vi "test_read-nmea-data2.vi"() -> ()   [LabVIEW 2019] (continued)
308,,2*7E\n\t\n15:10:22.66\tF9P\t$GBGSV,1,1,03,11,50,131,19,14,87,138,20,33,60,219,20,1*47\n\t\n15:10:22.68\tF9P\t$GBGSV,1,1,03,11,50,131,,14,87,138,22,33,60,219,,3*4D\n\t\n15:10:22.70\tF9P\t$GNGLL,3723.57293,N,12656.88370,E,061024.00,A,A*7B\n\t\n15:10:22.72\tF9P\t\t\n15:10:22.74\tF9P\t\t\n15:10:22.76\tF9P\t\t\n15:10:22.78\tF9P\t\t\n15:10:22.80\tF9P\t\t\n15:10:22.82\tF9P\t\t\n15:10:22.84\tF9P\t\t\n15:10:22.86\tF9P\t\t\n15:10:22.88\tF9P\t\t\n15:10:22.90\tF9P\t\t\n15:10:22.92\tF9P\t\t\n15:10:22.94\tF9P\t\t\n15:10:22.96\tF9P\t\t\n15:10:22.98\tF9P\t\t\n15:10:23.00\tF9P\t\t\n15:10:23.02\tF9P\t\t\n15:10:23.04\tF9P\t\t\n15:10:23.06\tF9P\t\t\n15:10:23.08\tF9P\t\t\n15:10:23.10\tF9P\t\t\n15:10:23.12\tF9P\t\t\n15:10:23.14\tF9P\t\t\n15:10:23.16\tF9P\t\t\n15:10:23.18\tF9P\t\t\n15:10:23.20\tF9P\t\t\n15:10:23.22\tF9P\t\t\n15:10:23.24\tF9P\t$GNRMC,061025.00,A,3723.57257,N,12656.88383,E,0.634,,250720,,,A,V*1E\n\t\n15:10:23.26\tF9P\t$GNVTG,,T,,M,0.634,N,1.174,K,A*3F\n\t\n15:10:23.28\tF9P\t$GNGGA,061025.00,3723.57257,N,12656.88383,E,1,12,0.64,59.6,M,18.5,M,,*7C\n\t\n15:10:23.30\tF9P\t$GNGSA,A,3,12,06,19,05,17,09,04,02,,,,,1.19,0.64,1.00,1*0A\n\t\n15:10:23.32\tF9P\t$GNGSA,A,3,85,71,84,,,,,,,,,,1.19,0.64,1.00,2*0F\n\t\n15:10:23.34\tF9P\t$GNGSA,A,3,36,19,11,04,09,12,,,,,,,1.19,0.64,1.00,3*0A\n\t\n15:10:23.36\tF9P\t$GNGSA,A,3,14,11,33,,,,,,,,,,1.19,0.64,1.00,4*0B\n\t\n15:10:23.38\tF9P\t$GPGSV,3,1,09,02,54,318,21,04,19,044,12,05,36,246,24,06,65,046,25,1*6C\n\t\n15:10:23.40\tF9P\t$GPGSV,3,2,09,09,45,075,26,12,24,278,19,17,34,153,21,19,53,156,23,1*6A\n\t\n15:10:23.42\tF9P\t$GPGSV,3,3,09,25,12,307,12,1*5E\n\t\n15:10:23.44\tF9P\t$GPGSV,3,1,09,02,54,318,,04,19,044,,05,36,246,18,06,65,046,15,6*67\n\t\n15:10:23.46\tF9P\t$GPGSV,3,2,09,09,45,075,,12,24,278,,17,34,153,,19,53,156,,6*63\n\t\n15:10:23.48\tF9P\t$GPGSV,3,3,09,25,12,307,,6*5A\n\t\n15:10:23.50\tF9P\t$GLGSV,2,1,08,69,12,031,,70,72,041,,71,51,205,17,72,03,209,,1*74\n\t\n15:10:23.52\tF9P\t$GLGSV,2,2,08,77,01,326,,84,20,122,09,85,70,065,19,86,36,330,,1*7A\n\t\n15:10:23.54\tF9P\t$GLGSV,2,1,08,69,12,031,,70,72,041,,71,51,205,18,72,03,209,,3*79\n\t\n15:10:23.56\tF9P\t$GLGSV,2,2,08,77,01,326,,84,20,122,09,85,70,065,19,86,36,330,,3*78\n\t\n15:10:23.58\tF9P\t$GAGSV,2,1,08,02,09,298,09,04,66,119,25,09,31,193,17,11,71,357,25,7*75\n\t\n15:10:23.60\tF9P\t$GAGSV,2,2,08,12,40,102,09,19,27,045,21,25,09,249,,36,25,308,13,7*73\n\t\n15:10:23.62\tF9P\t$GAGSV,2,1,08,02,09,298,,04,66,119,,09,31,193,19,11,71,357,11,2*77\n\t\n15:10:23.64\tF9P\t$GAGSV,2,2,08,12,40,102,,19,27,045,,25,09,249,,36,25,308,,2*7E\n\t\n15:10:23.66\tF9P\t$GBGSV,1,1,03,11,50,131,19,14,87,138,21,33,60,219,21,1*47\n\t\n15:10:23.68\tF9P\t$GBGSV,1,1,03,11,50,131,,14,87,138,23,33,60,219,,3*4C\n\t\n15:10:23.70\tF9P\t$GNGLL,3723.57257,N,12656.88383,E,061025.00,A,A*7E\n\t\n15:10:23.72\tF9P\t\t\n15:10:23.74\tF9P\t\t\n15:10:23.76\tF9P\t\t\n15:10:23.78\tF9P\t\t\n15:10:23.80\tF9P\t\t\n15:10:23.82\tF9P\t\t\n15:10:23.84\tF9P\t\t\n15:10:23.86\tF9P\t\t\n15:10:23.88\tF9P\t\t\n15:10:23.90\tF9P\t\t\n15:10:23.92\tF9P\t\t\n15:10:23.95\tF9P\t\t\n15:10:23.97\tF9P\t\t\n15:10:23.99\tF9P\t\t\n15:10:24.01\tF9P\t\t\n15:10:24.03\tF9P\t\t\n15:10:24.05\tF9P\t\t\n15:10:24.07\tF9P\t\t\n15:10:24.09\tF9P\t\t\n15:10:24.11\tF9P\t\t\n15:10:24.13\tF9P\t\t\n15:10:24.15\tF9P\t\t\n15:10:24.17\tF9P\t\t\n15:10:24.19\tF9P\t\t\n15:10:24.21\tF9P\t\t\n15:10:24.23\tF9P\t\t\n15:10:24.25\tF9P\t$GNRMC,061026.00,A,3723.57217,N,12656.88385,E,0.897,,250720,,,A,V*18\n\t\n15:10:24.27\tF9P\t$GNVTG,,T,,M,0.897,N,1.661,K,A*3B\n\t\n15:10:24.29\tF9P\t$GNGGA,061026.00,3723.57217,N,12656.88385,E,1,12,0.64,59.8,M,18.5,M,,*73\n\t\n15:10:24.31\tF9P\t$GNGSA,A,3,12,06,19,05,17,09,04,02,,,,,1.19,0.64,1.00,1*0A\n\t\n15:10:24.33\tF9P\t$GNGSA,A,3,85,71,84,,,,,,,,,,1.19,0.64,1.00,2*0F\n\t\n15:10:24.35\tF9P\t$GNGSA,A,3,36,19,11,04,09,12,,,,,,,1.19,0.64,1.00,3*0A\n\t\n15:10:24.37\tF9P\t$GNGSA,A,3,14,11,33,,,,,,,,,,1.19,0.64,1.00,4*0B\n\t\n15:10:24.39\tF9P\t$GPGSV,3,1,09,02,54,318,23,04,19,044,11,05,36,246,25,06,65,046,30,1*68\n\t\n15:10:24.41\tF9P\t$GPGSV,3,2,09,09,45,075,27,12,24,278,20,17,34,153,24,19,53,156,21,1*66\n\t\n15:10:24.43\tF9P\t$GPGSV,3,3,09,25,12,307,13,1*5F\n\t\n15:10:24.45\tF9P\t$GPGSV,3,1,09,02,54,318,,04,19,044,,05,36,246,17,06,65,046,16,6*6B\n\t\n15:10:24.47\tF9P\t$GPGSV,3,2,09,09,45,075,19,12,24,278,,17,34,153,,19,53,156,,6*6B\n\t\n15:10:24.49\tF9P\t$GPGSV,3,3,09,25,12,307,,6*5A\n\t\n15:10:24.51\tF9P\t$GLGSV,2,1,08,69,12,031,,70,72,041,,71,51,205,16,72,03,209,,1*75\n\t\n15:10:24.53\tF9P\t$GLGSV,2,2,08,77,01,326,,84,20,122,09,85,70,065,19,86,36,330,,1*7A\n\t\n15:10:24.55\tF9P\t$GLGSV,2,1,08,69,12,031,,70,72,041,,71,51,205,18,72,03,209,,3*79\n\t\n15:10:24.57\tF9P\t$GLGSV,2,2,08,77,01,326,,84,20,122,10,85,70,065,19,86,36,330,,3*70\n\t\n15:10:24.59\tF9P\t$GAGSV,2,1,08,02,09,298,09,04,66,119,25,09,31,193,18,11,71,357,25,7*7A\n\t\n15:10:24.61\tF9P\t$GAGSV,2,2,08,12,40,102,10,19,27,045,20,25,09,249,,36,25,308,13,7*7A\n\t\n15:10:24.63\tF9P\t$GAGSV,2,1,08,02,09,298,,04,66,119,,09,31,193,20,11,71,357,09,2*74\n\t\n15:10:24.65\tF9P\t$GAGSV,2,2,08,12,40,102,,19,27,045,,25,09,249,,36,25,308,,2*7E\n\t\n15:10:24.67\tF9P\t$GBGSV,1,1,03,11,50,131,21,14,87,138,20,33,60,219,20,1*4C\n\t\n15:10:24.69\tF9P\t$GBGSV,1,1,03,11,50,131,,14,87,138,23,33,60,219,,3*4C\n\t\n15:10:24.71\tF9P\t$GNGLL,3723.57217,N,12656.88385,E,061026.00,A,A*7F\n\t\n15:10:24.73\tF9P\t\t\n15:10:24.75\tF9P\t\t\n15:10:24.77\tF9P\t\t\n15:10:24.79\tF9P\t\t\n15:10:24.81\tF9P\t\t\n15:10:24.83\tF9P\t\t\n15:10:24.85\tF9P\t\t\n15:10:24.87\tF9P\t\t\n15:10:24.89\tF9P\t\t\n15:10:24.91\tF9P\t\t\n15:10:24.93\tF9P\t\t\n15:10:24.95\tF9P\t\t\n15:10:24.97\tF9P\t\t\n15:10:24.99\tF9P\t\t\n15:10:25.01\tF9P\t\t\n15:10:25.03\tF9P\t\t\n15:10:25.05\tF9P\t\t\n15:10:25.07\tF9P\t\t\n15:10:25.09\tF9P\t\t\n15:10:25.11\tF9P\t\t\n15:10:25.13\tF9P\t\t\n15:10:25.15\tF9P\t\t\n15:10:25.17\tF9P\t\t\n15:10:25.19\tF9P\t\t\n15:10:25.21\tF9P\t\t\n15:10:25.23\tF9P\t\t\n15:10:25.25\tF9P\t$GNRMC,061027.00,A,3723.57149,N,12656.88411,E,2.245,169.19,250720,,,A,V*04\n\t\n15:10:25.27\tF9P\t$GNVTG,169.19,T,,M,2.245,N,4.158,K,A*2C\n\t\n15:10:25.29\tF9P\t$GNGGA,061027.00,3723.57149,N,12656.88411,E,1,12,0.64,59.6,M,18.5,M,,*7E\n\t\n15:10:25.31\tF9P\t$GNGSA,A,3,12,06,19,05,17,09,04,02,,,,,1.19,0.64,1.00,1*0A\n\t\n15:10:25.33\tF9P\t$GNGSA,A,3,85,71,84,,,,,,,,,,1.19,0.64,1.00,2*0F\n\t\n15:10:25.35\tF9P\t$GNGSA,A,3,36,19,11,04,09,12,,,,,,,1.19,0.64,1.00,3*0A\n\t\n15:10:25.37\tF9P\t$GNGSA,A,3,14,11,33,,,,,,,,,,1.19,0.64,1.00,4*0B\n\t\n15:10:25.39\tF9P\t$GPGSV,3,1,09,02,54,318,23,04,19,044,08,05,36,246,26,06,65,046,22,1*60\n\t\n15:10:25.41\tF9P\t$GPGSV,3,2,09,09,45,075,26,12,24,278,23,17,34,153,23,19,53,156,22,1*60\n\t\n15:10:25.43\tF9P\t$GPGSV,3,3,09,25,12,307,14,1*58\n\t\n15:10:25.45\tF9P\t$GPGSV,3,1,09,02,54,318,,04,19,044,,05,36,246,19,06,65,046,16,6*65\n\t\n15:10:25.47\tF9P\t$GPGSV,3,2,09,09,45,075,18,12,24,278,,17,34,153,20,19,53,156,,6*68\n\t\n15:10:25.49\tF9P\t$GPGSV,3,3,09,25,12,307,,6*5A\n\t\n15:10:25.51\tF9P\t$GLGSV,2,1,08,69,12,031,,70,72,041,,71,51,205,16,72,03,209,,1*75\n\t\n15:10:25.53\tF9P\t$GLGSV,2,2,08,77,01,326,,84,20,122,12,85,70,065,20,86,36,330,,1*7A\n\t\n15:10:25.55\tF9P\t$GLGSV,2,1,08,69,12,031,,70,72,041,,71,51,205,18,72,03,209,,3*79\n\t\n15:10:25.57\tF9P\t$GLGSV,2,2,08,77,01,326,,84,20,122,09,85,70,065,18,86,36,330,,3*79\n\t\n15:10:25.59\tF9P\t$GAGSV,2,1,08,02,09,298,07,04,66,119,26,09,31,193,17,11,71,357,25,7*78\n\t\n15:10:25.61\tF9P\t$GAGSV,2,2,08,12,40,102,12,19,27,045,21,25,09,249,,36,25,308,13,7*79\n\t\n15:10:25.63\tF9P\t$GAGSV,2,1,08,02,09,298,,04,66,119,,09,31,193,19,11,71,357,08,2*7F\n\t\n15:10:25.65\tF9P\t$GAGSV,2,2,08,12,40,102,,19,27,045,,25,09,249,,36,25,308,,2*7E\n\t\n15:10:25.67\tF9P\t$GBGSV,1,1,03,11,50,131,22,14,87,138,22,33,60,219,21,1*4C\n\t\n15:10:25.69\tF9P\t$GBGSV,1,1,03,11,50,131,,14,87,138,22,33,60,219,,3*4D\n\t\n15:10:25.71\tF9P\t$GNGLL,3723.57149,N,12656.88411,E,061027.00,A,A*7C\n\t\n15:10:25.73\tF9P\t\t\n15:10:25.75\tF9P\t\t\n15:10:25.77\tF9P\t\t\n15:10:25.79\tF9P\t\t\n15:10:25.81\tF9P\t\t\n15:10:25.83\tF9P\t\t\n15:10:25.85\tF9P\t\t\n15:10:25.87\tF9P\t\t\n15:10:25.89\tF9P\t\t\n15:10:25.91\tF9P\t\t\n15:10:25.93\tF9P\t\t\n15:10:25.95\tF9P\t\t\n15:10:25.97\tF9P\t\t\n15:10:25.99\tF9P\t\t\n15:10:26.01\tF9P\t\t\n15:10:26.03\tF9P\t\t\n15:10:26.05\tF9P\t\t\n15:10:26.07\tF9P\t\t\n15:10:26.09\tF9P\t\t\n15:10:26.11\tF9P\t\t\n15:10:26.13\tF9P\t\t\n15:10:26.15\tF9P\t\t\n15:10:26.17\tF9P\t\t\n15:10:26.19\tF9P\t\t\n15:10:26.21\tF9P\t\t\n15:10:26.23\tF9P\t\t\n15:10:26.25\tF9P\t$GNRMC,061028.00,A,3723.57082,N,12656.88425,E,1.515,,250720,,,A,V*13\n\t\n15:10:26.27\tF9P\t$GNVTG,,T,,M,1.515,N,2.806,K,A*31\n\t\n15:10:26.29\tF9P\t$GNGGA,061028.00,3723.57082,N,12656.88425,E,1,12,0.64,61.5,M,18.5,M,,*78\n\t\n15:10:26.31\tF9P\t$GNGSA,A,3,12,06,19,05,17,09,04,02,,,,,1.18,0.64,1.00,1*0B\n\t\n15:10:26.33\tF9P\t$GNGSA,A,3,85,71,84,,,,,,,,,,1.18,0.64,1.00,2*0E\n\t\n15:10:26.35\tF9P\t$GNGSA,A,3,36,19,11,04,09,12,,,,,,,1.18,0.64,1.00,3*0B\n\t\n15:10:26.37\tF9P\t$GNGSA,A,3,14,11,33,,,,,,,,,,1.18,0.64,1.00,4*0A\n\t\n15:10:26.39\tF9P\t$GPGSV,3,1,09,02,54,318,22,04,19,044,12,05,36,246,26,06,65,046,23,1*6B\n\t\n15:10:26.41\tF9P\t$GPGSV,3,2,09,09,45,075,25,12,24,278,22,17,34,153,23,19,53,156,23,1*63\n\t\n15:10:26.43\tF9P\t$GPGSV,3,3,09,25,12,307,12,1*5E\n\t\n15:10:26.45\tF9P\t$GPGSV,3,1,09,02,54,318,,04,19,044,,05,36,246,19,06,65,046,15,6*66\n\t\n15:10:26.47\tF9P\t$GPGSV,3,2,09,09,45,075,17,12,24,278,,17,34,153,19,19,53,156,,6*6D\n\t\n15:10:26.49\tF9P\t$GPGSV,3,3,09,25,12,307,,6*5A\n\t\n15:10:26.51\tF9P\t$GLGSV,2,1,08,69,12,031,,70,72,041,,71,51,205,15,72,03,209,,1*76\n\t\n15:10:26.53\tF9P\t$GLGSV,2,2,08,77,01,326,,84,20,122,09,85,70,065,22,86,36,330,,1*72\n\t\n15:10:26.55\tF9P\t$GLGSV,2,1,08,69,12,031,,70,72,041,,71,51,205,17,72,03,209,,3*76\n\t\n15:10:26.57\tF9P\t$GLGSV,2,2,08,77,01,326,,84,20,122,13,85,70,065,18,86,36,330,,3*72\n\t\n15:10:26.59\tF9P\t$GAGSV,2,1,08,02,09,298,10,04,66,119,24,09,31,193,17,11,71,357,25,7*7C\n\t\n15:10:26.61\tF9P\t$GAGSV,2,2,08,12,40,102,13,19,27,045,28,25,09,249,,36,25,308,12,7*70\n\t\n15:10:26.63\tF9P\t$GAGSV,2,1,08,02,09,298,,04,66,119,,09,31,193,19,11,71,357,,2*77\n\t\n15:10:26.65\tF9P\t$GAGSV,2,2,08,12,40,102,,19,27,045,,25,09,249,,36,25,308,,2*7E\n\t\n15:10:26.67\tF9P\t$GBGSV,1,1,03,11,50,131,21,14,87,138,21,33,60,219,21,1*4C\n\t\n15:10:26.69\tF9P\t$GBGSV,1,1,03,11,50,131,,14,87,138,22,33,60,219,,3*4D\n\t\n15:10:26.71\tF9P\t$GNGLL,3723.57082,N,12656.88425,E,061028.00,A,A*72\n\t\n15:10:26.73\tF9P\t\t\n15:10:26.75\tF9P\t\t\n15:10:26.77\tF9P\t\t\n15:10:26.79\tF9P\t\t\n15:10:26.81\tF9P\t\t\n15:10:26.83\tF9P\t\t\n15:10:26.85\tF9P\t\t\n15:10:26.87\tF9P\t\t\n15:10:26.89\tF9P\t\t\n15:10:26.91\tF9P\t\t\n15:10:26.93\tF9P\t\t\n15:10:26.95\tF9P\t\t\n15:10:26.97\tF9P\t\t\n15:10:26.99\tF9P\t\t\n15:10:27.01\tF9P\t\t\n15:10:27.03\tF9P\t\t\n15:10:27.05\tF9P\t\t\n15:10:27.07\tF9P\t\t\n15:10:27.09\tF9P\t\t\n15:10:27.11\tF9P\t\t\n15:10:27.13\tF9P\t\t\n15:10:27.15\tF9P\t\t\n15:10:27.17\tF9P\t\t\n15:10:27.19\tF9P\t\t\n15:10:27.21\tF9P\t\t\n15:10:27.23\tF9P\t\t\n15:10:27.25\tF9P\t$GNRMC,061029.00,A,3723.57008,N,12656.88462,E,2.453,165.29,250720,,,A,V*04\n\t\n15:10:27.27\tF9P\t$GNVTG,165.29,T,,M,2.453,N,4.543,K,A*2C\n\t\n15:10:27.29\tF9P\t$GNGGA,061029.00,3723.57008,N,12656.88462,E,1,12,0.64,62.2,M,18.5,M,,*7C\n\t\n15:10:27.31\tF9P\t$GNGSA,A,3,12,06,19,05,17,09,04,02,,,,,1.18,0.64,1.00,1*0B\n\t\n15:10:27.33\tF9P\t$GNGSA,A,3,85,71,84,,,,,,,,,,1.18,0.64,1.00,2*0E\n\t\n15:10:27.35\tF9P\t$GNGSA,A,3,36,19,11,04,09,12,,,,,,,1.18,0.64,1.00,3*0B\n\t\n15:10:27.37\tF9P\t$GNGSA,A,3,14,11,33,,,,,,,,,,1.18,0.64,1.00,4*0A\n\t\n15:10:27.39\tF9P\t$GPGSV,3,1,09,02,54,318,23,04,19,044,15,05,36,246,24,06,65,046,24,1*68\n\t\n15:10:27.41\tF9P\t$GPGSV,3,2,09,09,45,075,24,12,24,278,21,17,34,153,23,19,53,156,23,1*61\n\t\n15:10:27.43\tF9P\t$GPGSV,3,3,09,25,12,307,13,1*5F\n\t\n15:10:27.45\tF9P\t$GPGSV,3,1,09,02,54,318,,04,19,044,,05,36,246,18,06,65,046,16,6*64\n\t\n15:10:27.47\tF9P\t$GPGSV,3,2,09,09,45,075,16,12,24,278,,17,34,153,17,19,53,156,,6*62\n\t\n15:10:27.49\tF9P\t$GPGSV,3,3,09,25,12,307,,6*5A\n\t\n15:10:27.51\tF9P\t$GLGSV,2,1,08,69,12,031,,70,72,041,,71,51,205,16,72,03,209,,1*75\n\t\n15:10:27.53\tF9P\t$GLGSV,2,2,08,77,01,326,,84,20,122,10,85,70,065,23,86,36,330,,1*7B\n\t\n15:10:27.55\tF9P\t$GLGSV,2,1,08,69,12,031,,70,72,041,,71,51,205,17,72,03,209,,3*76\n\t\n15:10:27.57\tF9P\t$GLGSV,2,2,08,77,01,326,,84,20,122,11,85,70,065,20,86,36,330,,3*7B\n\t\n15:10:27.59\tF9P\t$GAGSV,2,1,08,02,09,298,08,04,66,119,23,09,31,193,18,11,71,357,25,7*7D\n\t\n15:10:27.61\tF9P\t$GAGSV,2,2,08,12,40,102,09,19,27,045,19,25,09,249,,36,25,308,12,7*79\n\t\n15:10:27.63\tF9P\t$GAGSV,2,1,08,02,09,298,,04,66,119,,09,31,193,18,11,71,357,,2*76\n\t\n15:10:27.65\tF9P\t$GAGSV,2,2,08,12,40,102,,19,27,045,,25,09,249,,36,25,308,,2*7E\n\t\n15:10:27.67\tF9P\t$GBGSV,1,1,03,11,50,131,21,14,87,138,20,33,60,219,21,1*4D\n\t\n15:10:27.69\tF9P\t$GBGSV,1,1,03,11,50,131,,14,87,138,21,33,60,219,,3*4E\n\t\n15:10:27.71\tF9P\t$GNGLL,3723.57008,N,12656.88462,E,061029.00,A,A*72\n\t\n15:10:27.73\tF9P\t\t\n15:10:27.75\tF9P\t\t\n15:10:27.77\tF9P\t\t\n15:10:27.79\tF9P\t\t\n15:10:27.81\tF9P\t\t\n15:10:27.83\tF9P\t\t\n15:10:27.85\tF9P\t\t\n15:10:27.87\tF9P\t\t\n15:10:27.89\tF9P\t\t\n15:10:27.91\tF9P\t\t\n15:10:27.93\tF9P\t\t\n15:10:27.95\tF9P\t\t\n15:10:27.97\tF9P\t\t\n15:10:27.99\tF9P\t\t\n15:10:28.01\tF9P\t\t\n15:10:28.03\tF9P\t\t\n15:10:28.05\tF9P\t\t\n15:10:28.07\tF9P\t\t\n15:10:28.09\tF9P\t\t\n15:10:28.11\tF9P\t\t\n15:10:28.13\tF9P\t\t\n15:10:28.15\tF9P\t\t\n15:10:28.17\tF9P\t\t\n15:10:28.19\tF9P\t\t\n15:10:28.21\tF9P\t\t\n15:10:28.23\tF9P\t\t\n15:10:28.25\tF9P\t$GNRMC,061030.00,A,3723.56903,N,12656.88505,E,3.403,166.35,250720,,,A,V*05\n\t\n15:10:28.27\tF9P\t$GNVTG,166.35,T,,M,3.403,N,6.302,K,A*27\n\t\n15:10:28.29\tF9P\t$GNGGA,061030.00,3723.56903,N,12656.88505,E,1,12,0.68,62.9,M,18.5,M,,*70\n\t\n15:10:28.31\tF9P\t$GNGSA,A,3,12,06,19,05,17,09,02,,,,,,1.28,0.68,1.08,1*08\n\t\n15:10:28.33\tF9P\t$GNGSA,A,3,85,71,84,,,,,,,,,,1.28,0.68,1.08,2*09\n\t\n15:10:28.35\tF9P\t$GNGSA,A,3,36,19,11,04,09,12,,,,,,,1.28,0.68,1.08,3*0C\n\t\n15:10:28.37\tF9P\t$GNGSA,A,3,14,11,33,,,,,,,,,,1.28,0.68,1.08,4*0D\n\t\n15:10:28.39\tF9P\t$GPGSV,3,1,09,02,54,318,23,04,18,044,,05,36,246,24,06,65,046,27,1*6E\n\t\n15:10:28.41\tF9P\t$GPGSV,3,2,09,09,45,075,22,12,24,278,20,17,34,153,22,19,53,156,23,1*67\n\t\n15:10:28.43\tF9P\t$GPGSV,3,3,09,25,12,307,10,1*5C\n\t\n15:10:28.45\tF9P\t$GPGSV,3,1,09,02,54,318,,04,18,044,,05,36,246,18,06,65,046,17,6*64\n\t\n15:10:28.47\tF9P\t$GPGSV,3,2,09,09,45,075,16,12,24,278,,17,34,153,15,19,53,156,,6*60\n\t\n15:10:28.49\tF9P\t$GPGSV,3,3,09,25,12,307,,6*5A\n\t\n15:10:28.51\tF9P\t$GLGSV,2,1,08,69,12,031,,70,72,041,,71,51,205,15,72,03,209,,1*76\n\t\n15:10:28.53\tF9P\t$GLGSV,2,2,08,77,01,326,,84,20,122,10,85,70,065,22,86,36,330,,1*7A\n\t\n15:10:28.55\tF9P\t$GLGSV,2,1,08,69,12,031,,70,72,041,,71,51,205,18,72,03,209,,3*79\n\t\n15:10:28.57\tF9P\t$GLGSV,2,2,08,77,01,326,,84,20,122,10,85,70,065,20,86,36,330,,3*7A\n\t\n15:10:28.59\tF9P\t$GAGSV,2,1,08,02,09,298,08,04,66,119,21,09,31,193,18,11,71,357,25,7*7F\n\t\n15:10:28.61\tF9P\t$GAGSV,2,2,08,12,40,102,09,19,27,045,20,25,09,249,,36,25,308,13,7*72\n\t\n15:10:28.63\tF9P\t$GAGSV,2,1,08,02,09,298,,04,66,119,,09,31,193,18,11,71,357,,2*76\n\t\n15:10:28.65\tF9P\t$GAGSV,2,2,08,12,40,102,,19,27,045,,25,09,249,,36,25,308,,2*7E\n\t\n15:10:28.67\tF9P\t$GBGSV,1,1,03,11,50,131,19,14,87,138,19,33,60,219,21,1*4C\n\t\n15:10:28.69\tF9P\t$GBGSV,1,1,03,11,50,131,,14,87,138,21,33,60,219,,3*4E\n\t\n15:10:28.71\tF9P\t$GNGLL,3723.56903,N,12656.88505,E,061030.00,A,A*79\n\t\n15:10:28.73\tF9P\t\t\n15:10:28.75\tF9P\t\t\n15:10:28.77\tF9P\t\t\n15:10:28.79\tF9P\t\t\n15:10:28.81\tF9P\t\t\n15:10:28.83\tF9P\t\t\n15:10:28.85\tF9P\t\t\n15:10:28.87\tF9P\t\t\n15:10:28.89\tF9P\t\t\n15:10:28.91\tF9P\t\t\n15:10:28.93\tF9P\t\t\n15:10:28.95\tF9P\t\t\n15:10:28.97\tF9P\t\t\n15:10:28.99\tF9P\t\t\n15:10:29.01\tF9P\t\t\n15:10:29.03\tF9P\t\t\n15:10:29.05\tF9P\t\t\n15:10:29.07\tF9P\t\t\n15:10:29.09\tF9P\t\t\n15:10:29.11\tF9P\t\t\n15:10:29.13\tF9P\t\t\n15:10:29.15\tF9P\t\t\n15:10:29.17\tF9P\t\t\n15:10:29.19\tF9P\t\t\n15:10:29.21\tF9P\t\t\n15:10:29.23\tF9P\t\t\n15:10:29.25\tF9P\t$GNRMC,061031.00,A,3723.56820,N,12656.88516,E,2.268,,250720,,,A,V*15\n\t\n15:10:29.27\tF9P\t$GNVTG,,T,,M,2.268,N,4.200,K,A*35\n\t\n15:10:29.29\tF9P\t$GNGGA,061031.00,3723.56820,N,12656.88516,E,1,12,0.68,62.8,M,18.5,M,,*72\n\t\n15:10:29.31\tF9P\t$GNGSA,A,3,12,06,19,05,17,09,02,,,,,,1.28,0.68,1.08,1*08\n\t\n15:10:29.33\tF9P\t$GNGSA,A,3,85,71,84,,,,,,,,,,1.28,0.68,1.08,2*09\n\t\n15:10:29.35\tF9P\t$GNGSA,A,3,36,19,11,04,09,12,,,,,,,1.28,0.68,1.08,3*0C\n\t\n15:10:29.37\tF9P\t$GNGSA,A,3,14,11,33,,,,,,,,,,1.28,0.68,1.08,4*0D\n\t\n15:10:29.39\tF9P\t$GPGSV,3,1,09,02,54,318,22,04,18,044,,05,37,247,24,06,65,046,28,1*60\n\t\n15:10:29.41\tF9P\t$GPGSV,3,2,09,09,45,075,21,12,24,278,19,17,34,153,23,19,53,156,22,1*6E\n\t\n15:10:29.43\tF9P\t$GPGSV,3,3,09,25,12,307,09,1*54\n\t\n15:10:29.45\tF9P\t$GPGSV,3,1,09,02,54,318,,04,18,044,,05,37,247,17,06,65,046,15,6*69\n\t\n15:10:29.47\tF9P\t$GPGSV,3,2,09,09,45,075,15,12,24,278,,17,34,153,16,19,53,156,,6*60\n\t\n15:10:29.49\tF9P\t$GPGSV,3,3,09,25,12,307,,6*5A\n\t\n15:10:29.51\tF9P\t$GLGSV,2,1,08,69,12,031,,70,72,041,,71,51,205,15,72,03,209,,1*76\n\t\n15:10:29.53\tF9P\t$GLGSV,2,2,08,77,01,326,,84,20,122,09,85,70,065,21,86,36,330,,1*71\n\t\n15:10:29.55\tF9P\t$GLGSV,2,1,08,69,12,031,,70,72,041,,71,51,205,17,72,03,209,,3*76\n\t\n15:10:29.57\tF9P\t$GLGSV,2,2,08,77,01,326,,84,20,122,12,85,70,065,20,86,36,330,,3*78\n\t\n15:10:29.59\tF9P\t$GAGSV,2,1,08,02,09,298,10,04,66,119,21,09,31,193,19,11,71,357,25,7*77\n\t\n15:10:29.61\tF9P\t$GAGSV,2,2,08,12,40,102,08,19,27,045,21,25,09,249,,36,25,308,12,7*73\n\t\n15:10:29.63\tF9P\t$GAGSV,2,1,08,02,09,298,,04,66,119,,09,31,193,17,11,71,357,,2*79\n\t\n15:10:29.65\tF9P\t$GAGSV,2,2,08,12,40,102,,19,27,045,,25,09,249,,36,25,308,,2*7E\n\t\n15:10:29.67\tF9P\t$GBGSV,1,1,03,11,50,131,19,14,87,138,19,33,60,219,21,1*4C\n\t\n15:10:29.69\tF9P\t$GBGSV,1,1,03,11,50,131,,14,87,138,21,33,60,219,,3*4E\n\t\n15:10:29.71\tF9P\t$GNGLL,3723.56820,N,12656.88516,E,061031.00,A,A*7A\n\t\n15:10:29.73\tF9P\t\t\n15:10:29.75\tF9P\t\t\n15:10:29.77\tF9P\t\t\n15:10:29.79\tF9P\t\t\n15:10:29.81\tF9P\t\t\n15:10:29.83\tF9P\t\t\n15:10:29.85\tF9P\t\t\n15:10:29.87\tF9P\t\t\n15:10:29.89\tF9P\t\t\n15:10:29.91\tF9P\t\t\n15:10:29.93\tF9P\t\t\n15:10:29.95\tF9P\t\t\n15:10:29.97\tF9P\t\t\n15:10:29.99\tF9P\t\t\n15:10:30.01\tF9P\t\t\n15:10:30.03\tF9P\t\t\n15:10:30.05\tF9P\t\t\n15:10:30.07\tF9P\t\t\n15:10:30.09\tF9P\t\t\n15:10:30.11\tF9P\t\t\n15:10:30.13\tF9P\t\t\n15:10:30.15\tF9P\t\t\n15:10:30.17\tF9P\t\t\n15:10:30.19\tF9P\t\t\n15:10:30.21\tF9P\t\t\n15:10:30.23\tF9P\t\t\n15:10:30.25\tF9P\t$GNRMC,061032.00,A,3723.56746,N,12656.88501,E,2.408,,250720,,,A,V*1F\n\t\n15:10:30.27\tF9P\t$GNVTG,,T,,M,2.408,N,4.459,K,A*3F\n\t\n15:10:30.29\tF9P\t$GNGGA,061032.00,3723.56746,N,12656.88501,E,1,12,0.68,63.0,M,18.5,M,,*71\n\t\n15:10:30.31\tF9P\t$GNGSA,A,3,12,06,19,05,17,09,02,,,,,,1.28,0.68,1.08,1*08\n\t\n15:10:30.33\tF9P\t$GNGSA,A,3,85,71,84,,,,,,,,,,1.28,0.68,1.08,2*09\n\t\n15:10:30.35\tF9P\t$GNGSA,A,3,36,19,11,04,09,12,,,,,,,1.28,0.68,1.08,3*0C\n\t\n15:10:30.37\tF9P\t$GNGSA,A,3,14,11,33,,,,,,,,,,1.28,0.68,1.08,4*0D\n\t\n15:10:30.39\tF9P\t$GPGSV,3,1,09,02,54,318,22,04,18,044,19,05,37,247,23,06,64,047,27,1*60\n\t\n15:10:30.41\tF9P\t$GPGSV,3,2,09,09,45,075,21,12,24,278,18,17,34,153,23,19,53,156,23,1*6E\n\t\n15:10:30.43\tF9P\t$GPGSV,3,3,09,25,12,307,08,1*55\n\t\n15:10:30.45\tF9P\t$GPGSV,3,1,09,02,54,318,,04,18,044,,05,37,247,16,06,64,047,15,6*68\n\t\n15:10:30.47\tF9P\t$GPGSV,3,2,09,09,45,075,15,12,24,278,,17,34,153,16,19,53,156,,6*60\n\t\n15:10:30.49\tF9P\t$GPGSV,3,3,09,25,12,307,,6*5A\n\t\n15:10:30.51\tF9P\t$GLGSV,2,1,08,69,12,031,,70,72,041,,71,51,205,15,72,03,209,,1*76\n\t\n15:10:30.53\tF9P\t$GLGSV,2,2,08,77,01,326,,84,20,122,07,85,70,065,21,86,36,330,,1*7F\n\t\n15:10:30.55\tF9P\t$GLGSV,2,1,08,69,12,031,,70,72,041,,71,51,205,17,72,03,209,,3*76\n\t\n15:10:30.57\tF9P\t$GLGSV,2,2,08,77,01,326,,84,20,
